vi "Filter resources by name.vi"(10 "filter text":string, 11 "fpga resources in":T1[](array[typedef]) {"fpga cd" format="%.0x"}) -> (2 "filtered resource names out":string[](array[string]), 3 "filtered resources out":T1[](array[typedef]) {"fpga cd" format="%.0x"})   [LabVIEW 2016, in "FPGA RM System Definition API.lvlib"]
uses:
  FPGA RM System Definition API.lvlib
  Types/resources.ctl
  <vilib>/NI Veristand/Custom Device API/Custom Device Item Ref.ctl
  Shared/Types/fpga resource.ctl
  Shared/Types/Channel Type.ctl
  <vilib>/NI VeriStand/Custom Device API/Custom Device API.lvlib
  Shared/FPGA RM Shared API.lvlib
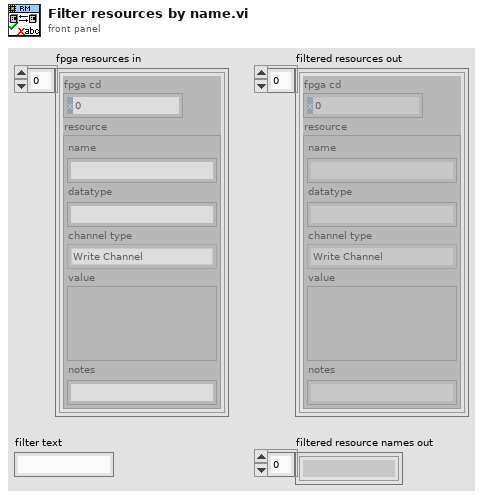
[diagram p1: front panel]
types:
  T1 = typedef "FPGA RM System Definition API.lvlib/resources.ctl" = cluster{"fpga cd":T2, "resource":T3}
  T2 = typedef "Custom Device API.lvlib/Custom Device Item Ref.ctl" = u64
  T3 = typedef "FPGA RM Shared API.lvlib/fpga resource.ctl" = cluster{"name":string, "datatype":string, "channel type":T4, "value":variant, "notes":string}
  T4 = typedef "FPGA RM Shared API.lvlib/Channel Type.ctl" = enum16{"Write Channel", "Read Channel", "Write Waveform", "Read Waveform"}
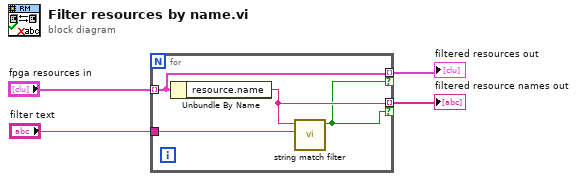
[diagram p0: block diagram]
diagram:
  n1 = for {
    tunnel: "fpga resources in" -> [w7] mode=indexing
    tunnel: "filter text" -> [w8]
    tunnel: [w7] -> w4 mode=indexing if=w5
    tunnel: [w6] -> w2 mode=indexing if=w5
    n2 = Unbundle By Name(w7) -> ("resource.name"=w6:string)
    n3 = call "string match filter.vi"("string filter value"=w8, "string value"=w6) -> ("match?"=w5:bool)  [unwired: 9 in]
  }
  "filtered resources out" <- w4
  "filtered resource names out" <- w2
